vi "field_sweep_0.vi"() -> ()   [LabVIEW 2016]
uses:
  states_field_sweep.ctl
  <vilib>/Utility/error.llb/DialogType.ctl
  <vilib>/DAQmx/write.llb/DAQmx Write (Analog DBL 1Chan 1Samp).vi
  <vilib>/DAQmx/create/channels.llb/DAQmx Create Channel (AO-Voltage-Basic).vi
  <vilib>/DAQmx/miscellaneous.llb/DAQmx Fill In Error Info.vi
  <instrlib>/niVNA/niVNA.llb/niVNA Fetch Sweep Measurement (DBL).vi
panel:
  out "DAQ channel Out":tag="DAQ_6363/ao0"
  in  "Averaging Points":i32=10 min=1 max=3201 step=1
  in  "DAQ channel In":tag="DAQ_6363/ao0"
  in  "Exit Button":bool
  in  "IF Bandwidth":dbl(ring)=1000.0 items=["10 Hz"=10.0, "30 Hz"=30.0, "100 Hz"=100.0, "300 Hz"=300.0, "1 KHz"=1000.0, "3 KHz"=3000.0, "10 KHz"=10000.0, "30 KHz"=30000.0]
  in  "Speed (Oe/sec)":dbl=5.0
  in  "Frequency (Hz)":dbl=3000000000.0 min=10000000.0 max=6000000000.0
  in  "Save Button":bool
  out "Status":string="Shutting down...Sweeping field to zero..."
  out "Cursor":cluster{"x":dbl, "y":dbl} {"x" format="%.2f"; "y" format="%.5f"}
  out "VNA Name Out":refnum<k15>="VNA_5630"
  out "Error Out":errorcluster
  in  "Error In (no error)":errorcluster
  in  "Format":i32(ring)=1 items=["Log Magnitude (dB)"=0, "Lin Magnitude"=1, "Phase (deg)"=2, "VSWR"=3, "Group Delay"=6]
  out "SpectrumGraph":cluster{"Field":dbl[], "Signal":dbl[]}(graph)
  in  "S-parameter":i32(ring)=1 caption="Measurement" items=["S11", "S21"]
  in  "Start Button":bool
  in  "Stop Button":bool
  in  "Output Power (dBm)":dbl=1.0 min=-25.0 max=5.0 step=0.5
  in  "Number of Points":i32=1000 min=1 max=3201 step=1
  in  "Stop H Field (Oe)":dbl=1500.0 min=-6000.0 max=6000.0 format="%#_6f"
  in  "Start H Field (Oe)":dbl=1000.0 min=-6000.0 max=6000.0 format="%#_6f"
  in  "VNA Name In":refnum<k15>="VNA_5630"
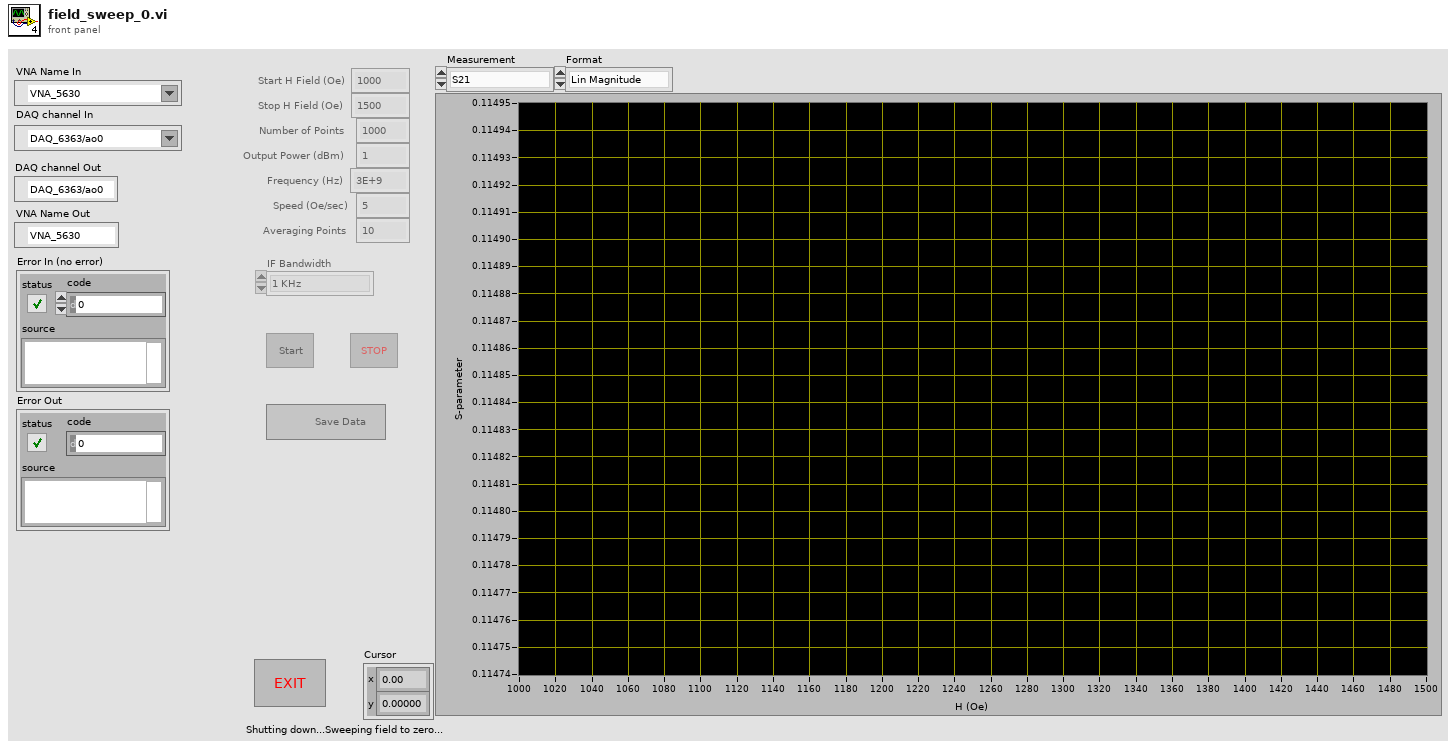
[diagram p1: front panel]
types:
  T1 = typedef "states_field_sweep.ctl" = enum16{"Init", "Idle", "Sweeping up", "Sweeping down", "Running", "Shutdown"}
  T2 = typedef "DialogType.ctl" = u16
  T3 = typedef "LVPoint32TypeDef.ctl" = cluster{"Horizontal":i32, "Vertical":i32}
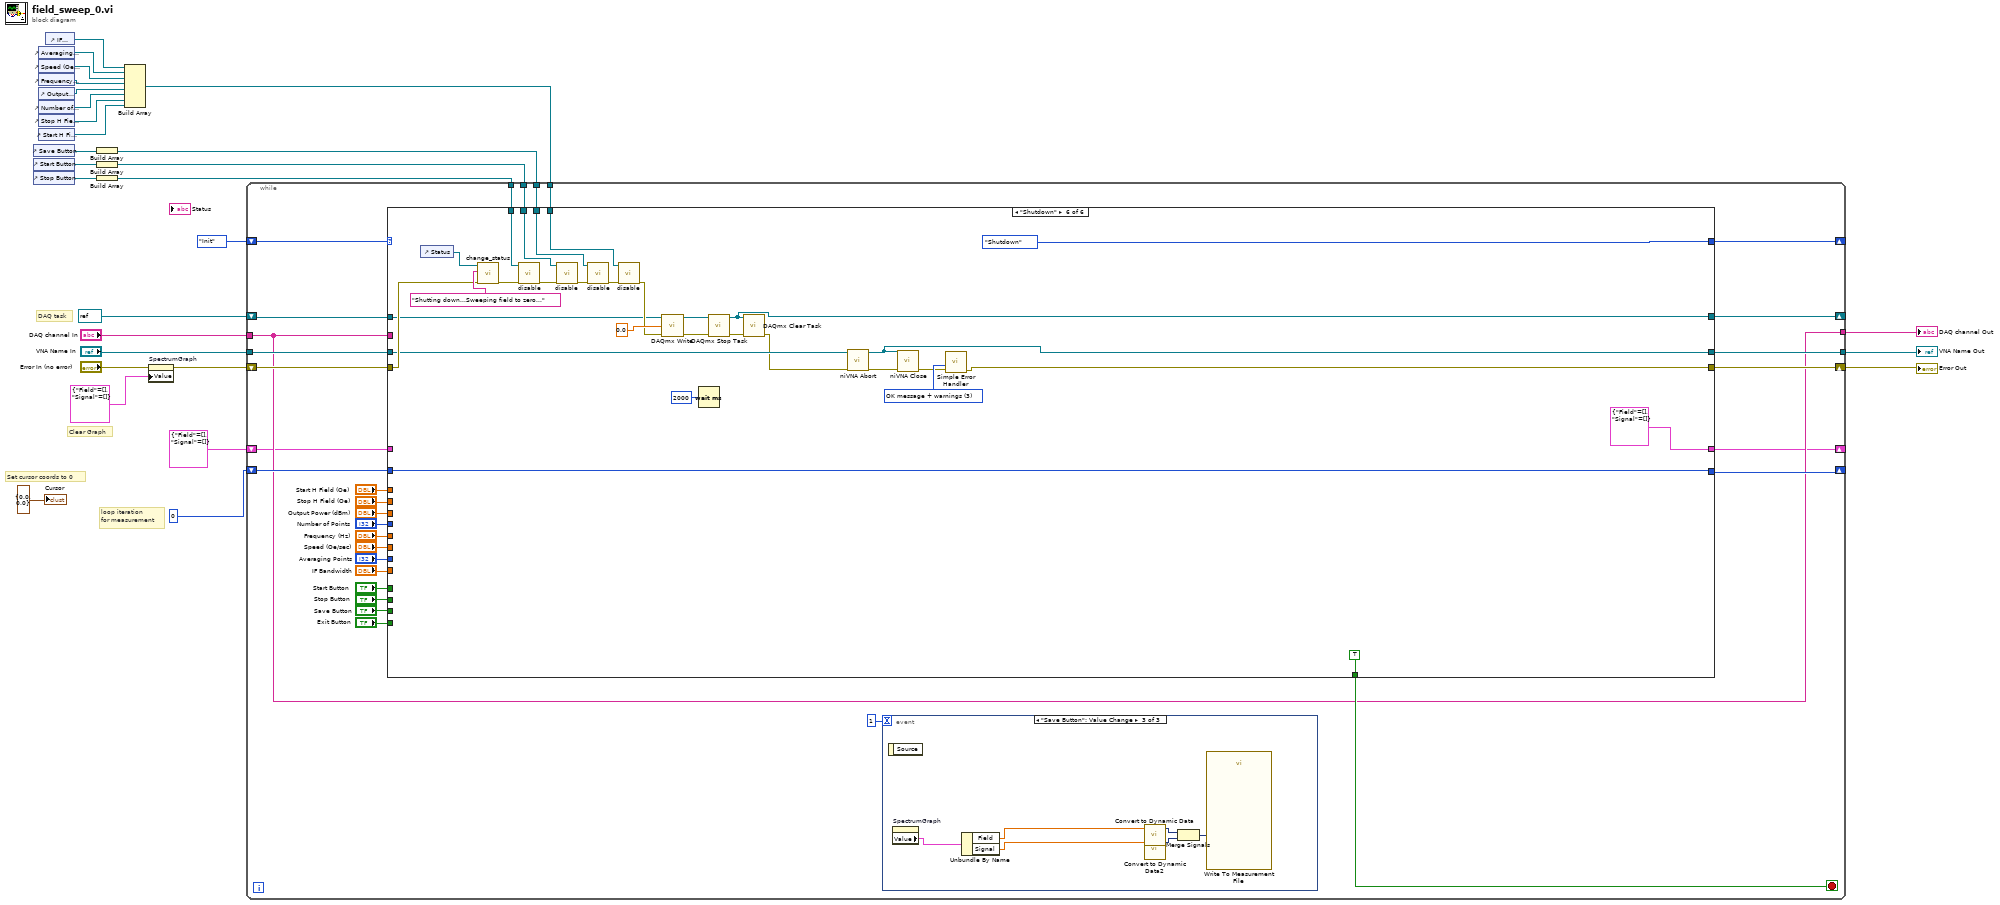
[diagram p0: block diagram]
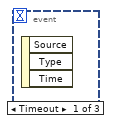
[diagram p2: hidden frame]
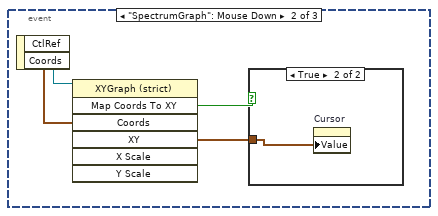
[diagram p3: hidden frame]
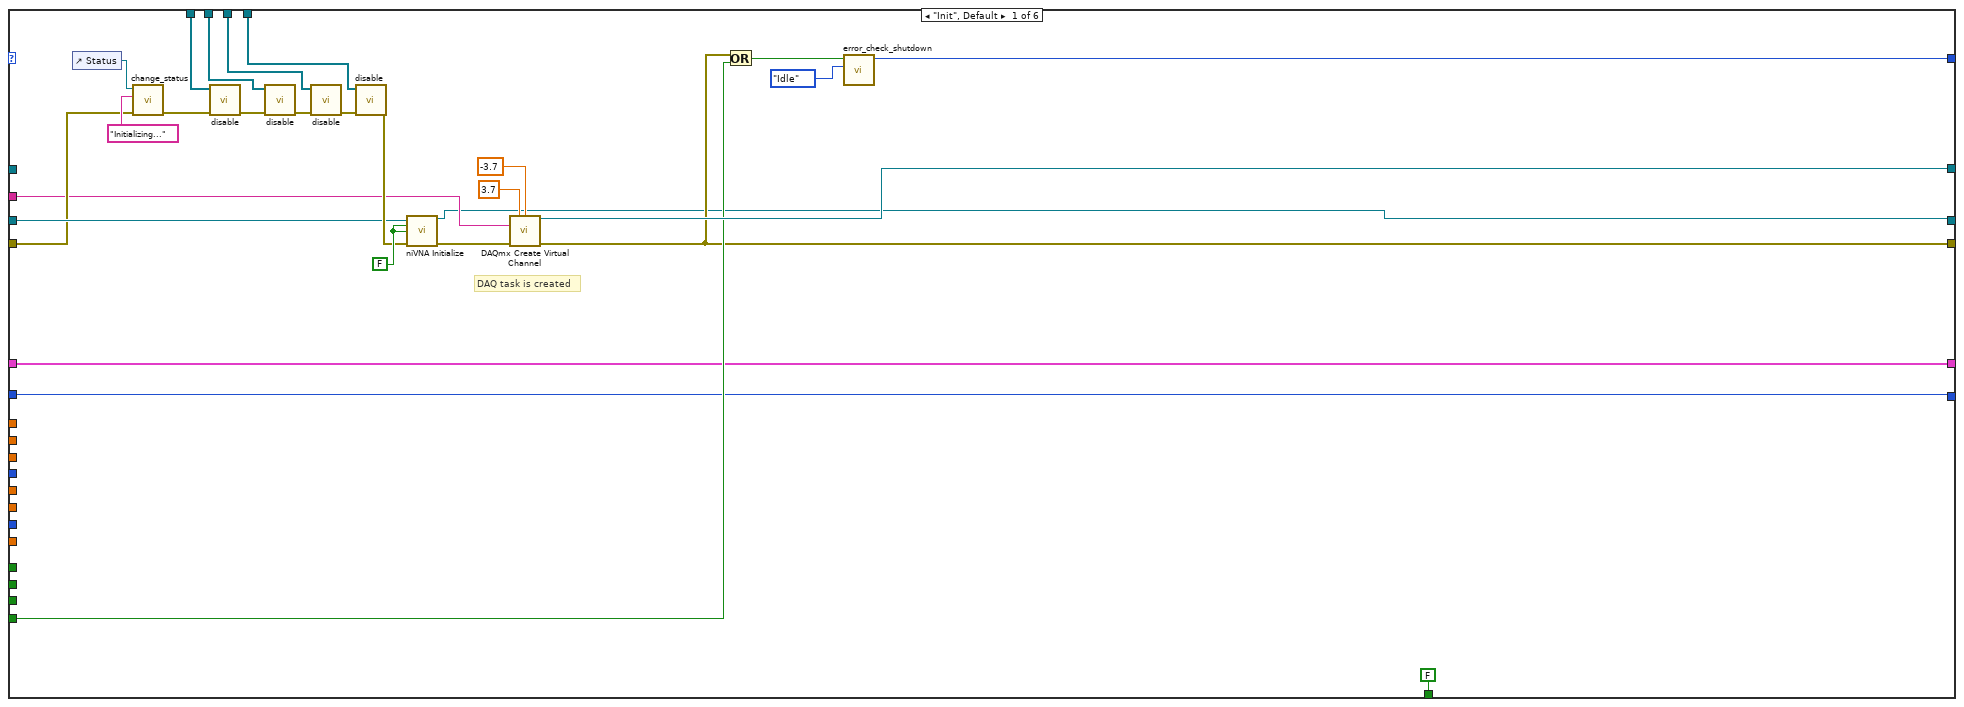
[diagram p5: hidden frame]
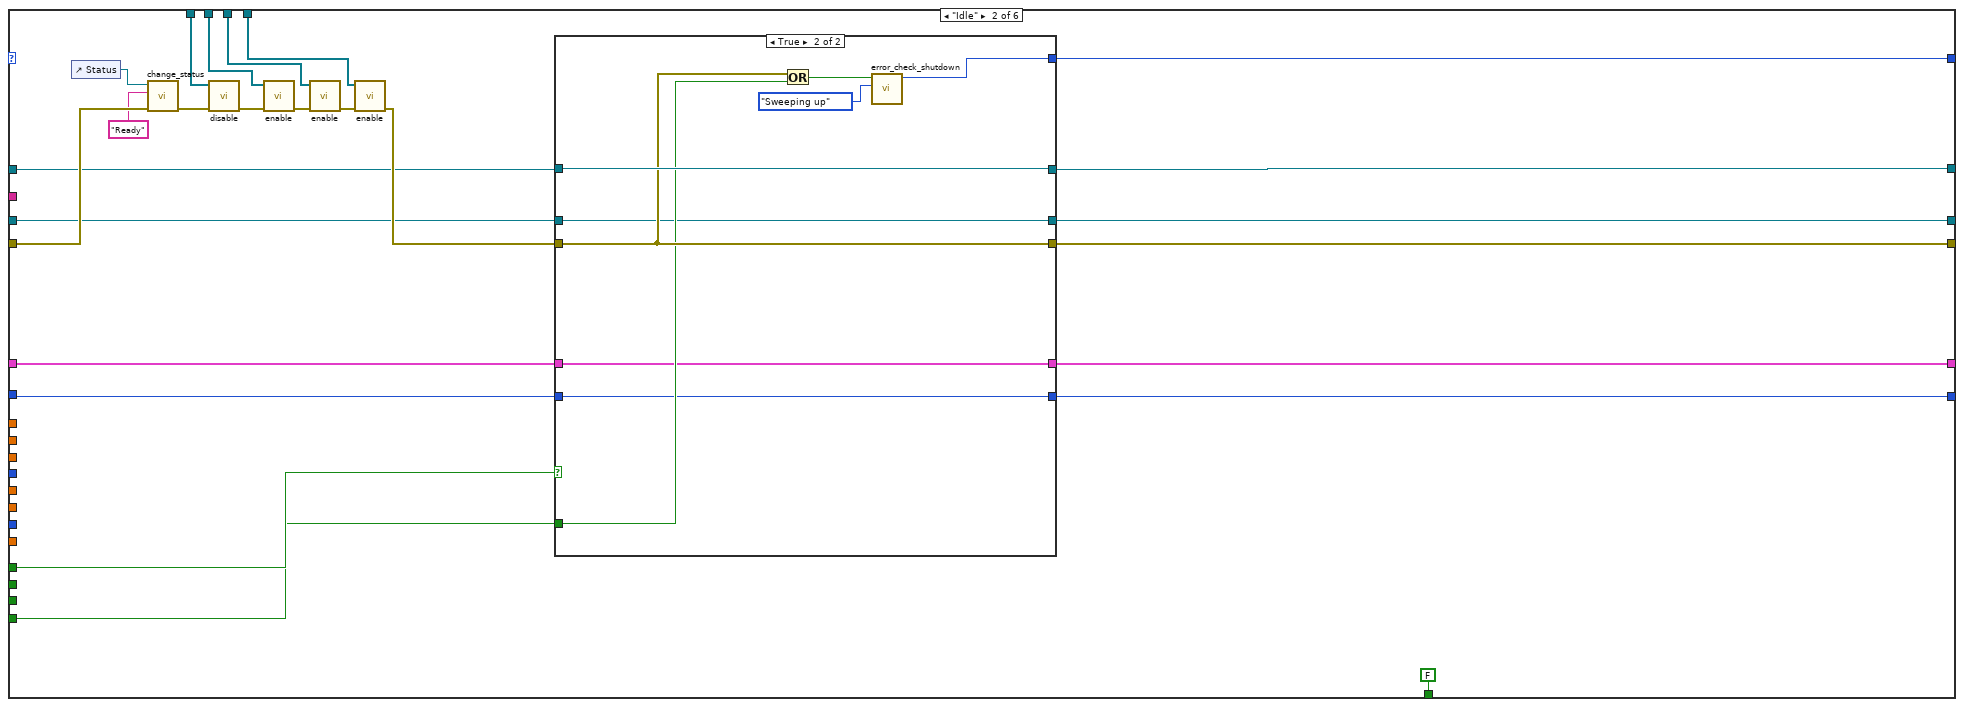
[diagram p6: hidden frame]
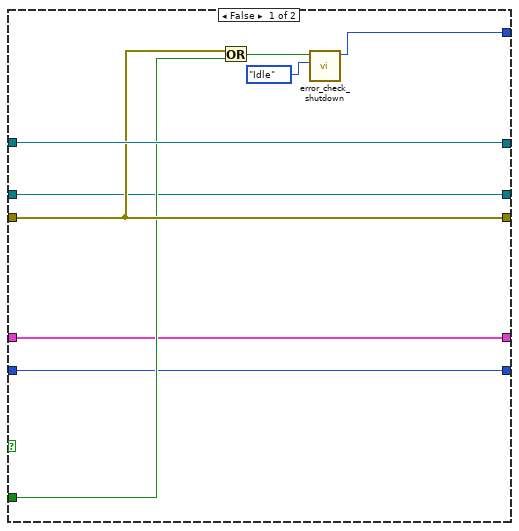
[diagram p7: hidden frame]
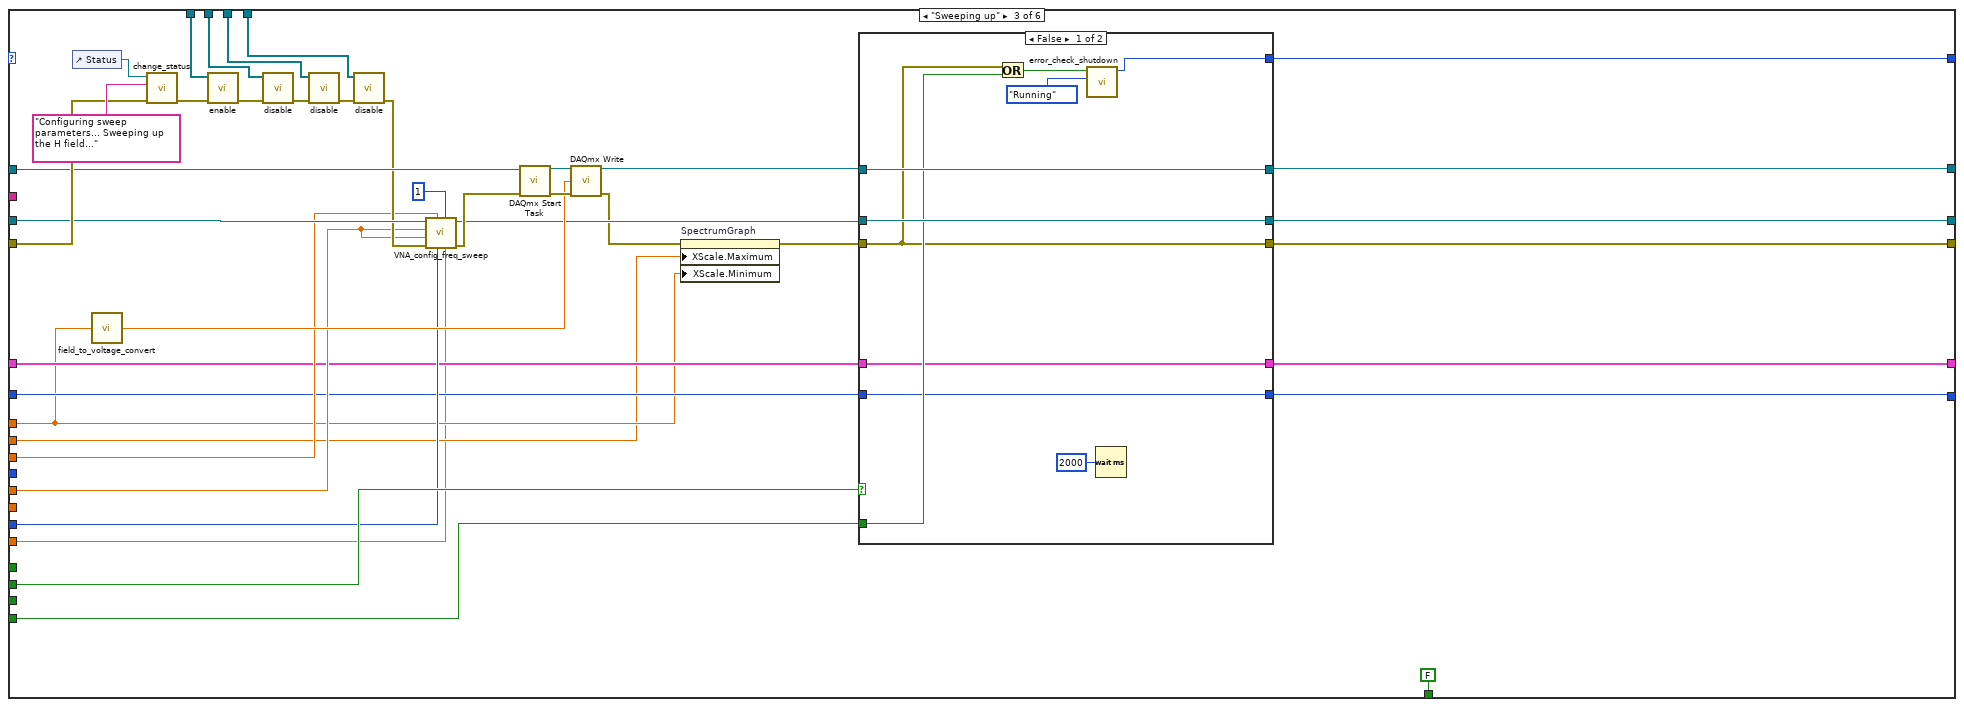
[diagram p8: hidden frame]
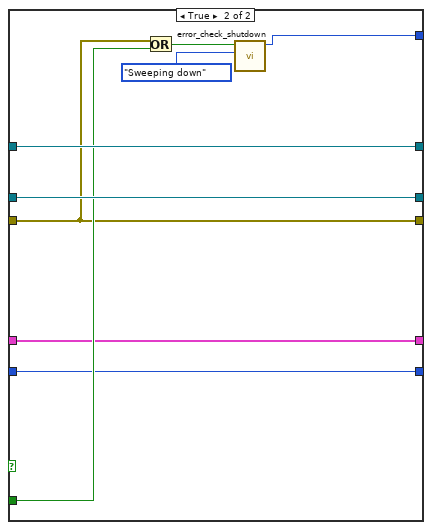
[diagram p9: hidden frame]
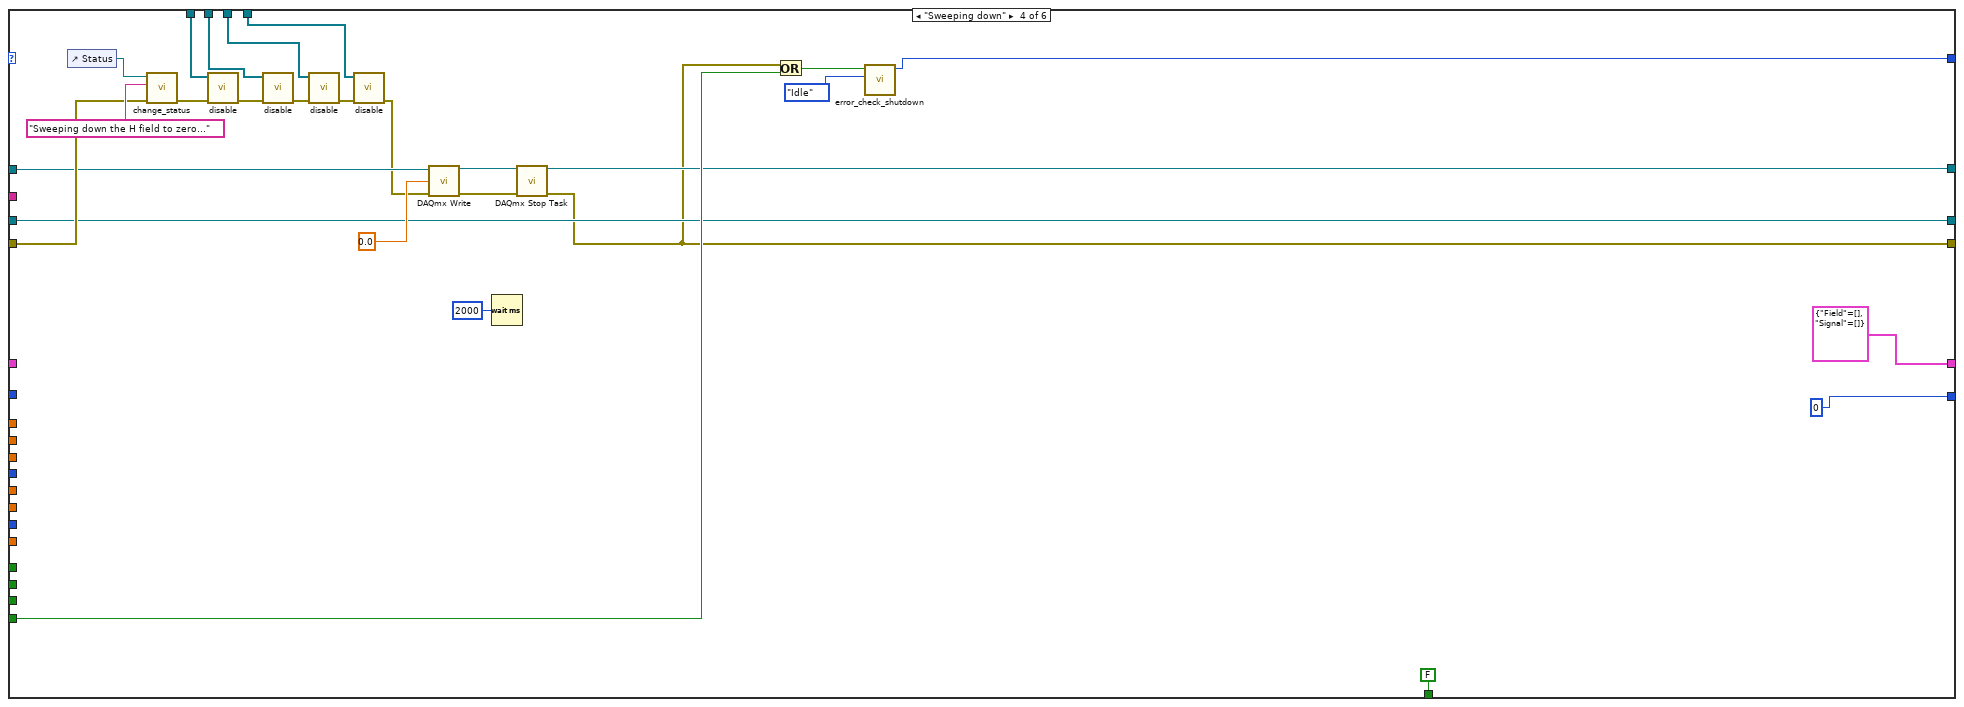
[diagram p10: hidden frame]
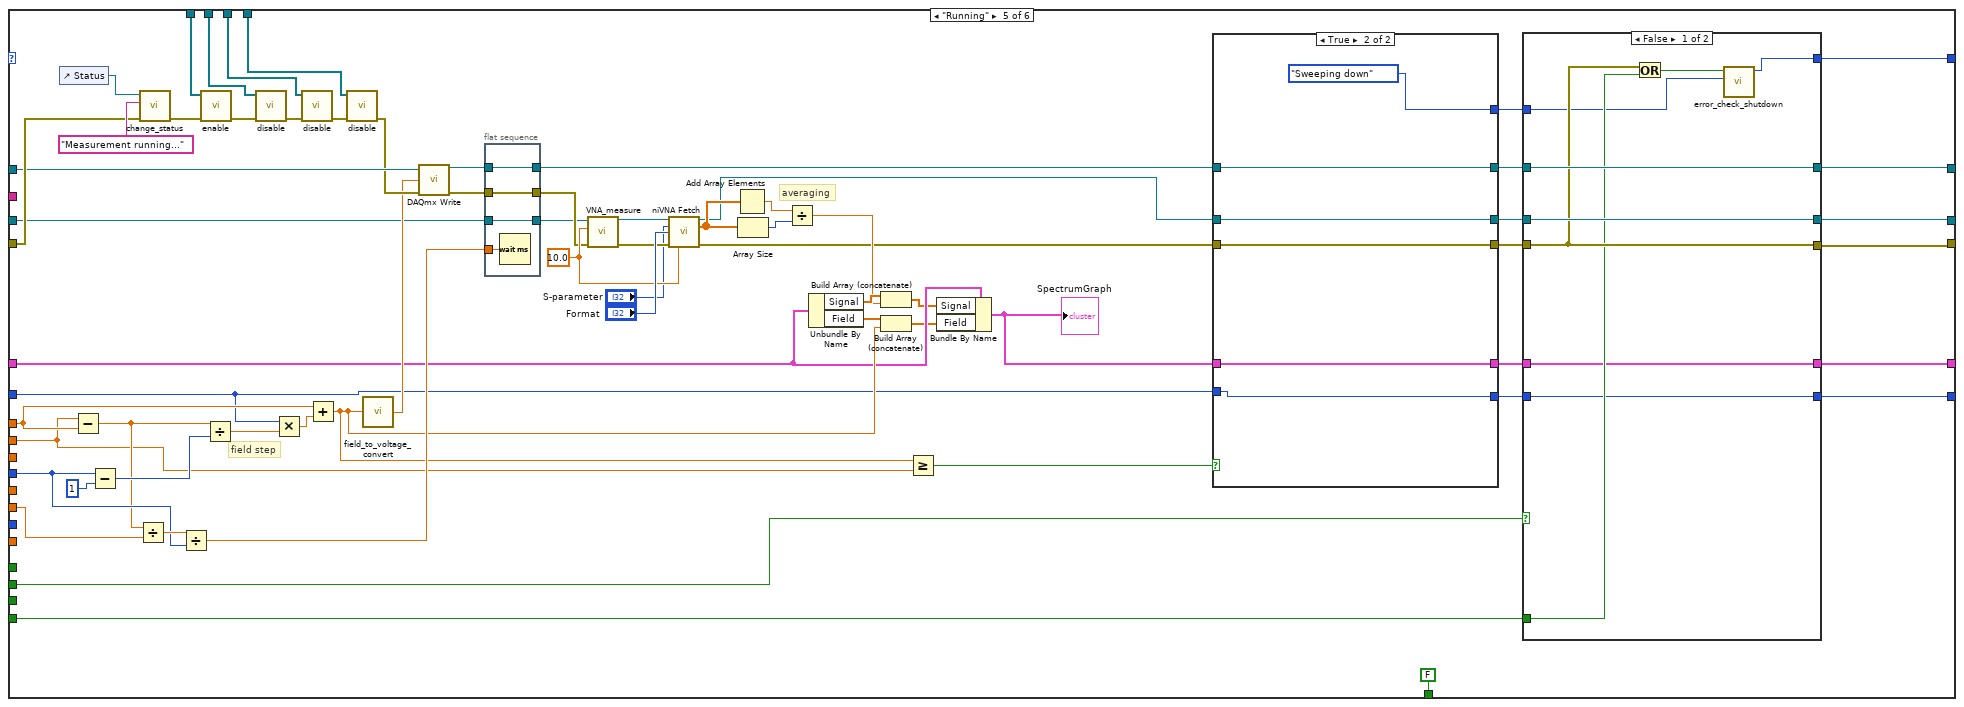
[diagram p11: hidden frame]
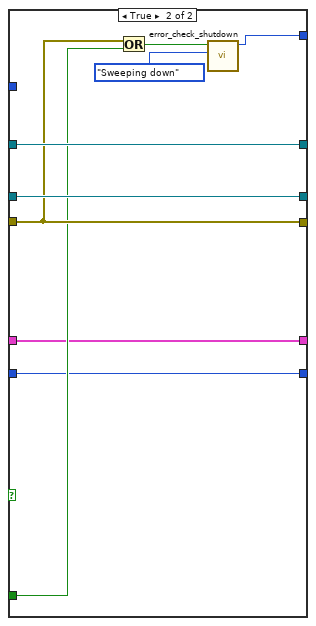
[diagram p12: hidden frame]
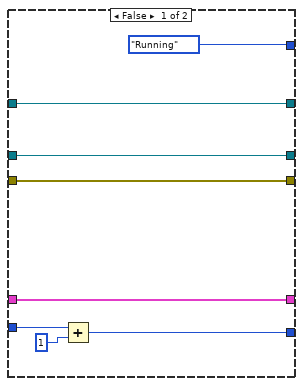
[diagram p13: hidden frame]
diagram:
  # "loop iteration\nfor measurement"
  # "DAQ task"
  # "Set cursor coords to 0"
  # "Clear Graph"
  n1 = control-ref of="Save Button"() -> (w11:refnum<vi>)
  n2 = control-ref of="Start Button"() -> (w19:refnum<vi>)
  n3 = control-ref of="Stop Button"() -> (w18:refnum<vi>)
  n4 = control-ref of="Averaging Points"() -> (w8:refnum<vi>)
  n5 = control-ref of="Speed (Oe/sec)"() -> (w25:refnum<vi>)
  n6 = control-ref of="Frequency (Hz)"() -> (w24:refnum<vi>)
  n7 = control-ref of="Output Power (dBm)"() -> (w23:refnum<vi>)
  n8 = control-ref of="Number of Points"() -> (w22:refnum<vi>)
  n9 = control-ref of="Stop H Field (Oe)"() -> (w21:refnum<vi>)
  n10 = control-ref of="Start H Field (Oe)"() -> (w20:refnum<vi>)
  n11 = control-ref of="IF Bandwidth"() -> (w26:refnum<vi>)
  n12 = Build Array(w11) -> (w10:refnum<vi>[])
  n13 = Build Array(w19) -> (w16:refnum<vi>[])
  n14 = Build Array(w18) -> (w15:refnum<vi>[])
  n15 = Build Array(w26, w8, w25, w24, w23, w22, w21, w20) -> (w17:refnum<vi>[])
  n16 = property on="SpectrumGraph" class="XYGraph (strict)"(error in="Error In (no error)", "Value"=cluster{"Field":dbl[], "Signal":dbl[]} {"Field"=[], "Signal"=[]} ("SpectrumGraph")) -> (error out=w3:errorcluster)  [unwired: 1 in, 1 out]
  n17 = while {
    shift-right: [w54] -> _
    shift-left: states_field_sweep."Init" -> [w59]
    shift-right: [w34] -> _
    shift-left: 0 -> [w36]
    tunnel: w17 -> [w58]
    tunnel: w16 -> [w57]
    tunnel: w15 -> [w56]
    tunnel: "VNA Name In" -> [w55]
    tunnel: "DAQ channel In" -> [w33]
    shift-right: [w53] -> w7
    shift-left: w3 -> [w52]
    shift-right: [w51] -> _
    shift-left: refnum<k21> refnum ("task in") -> [w50]
    tunnel: w10 -> [w49]
    tunnel: [w37] -> w6
    shift-right: [w29] -> _
    shift-left: cluster{"Field":dbl[], "Signal":dbl[]} {"Field"=[], "Signal"=[]} -> [w30]
    tunnel: [w33] -> w5
    stop <- w44 stop-if-true
    n18 = case shown="\"Shutdown\"" w59 {
      tunnel: w58 -> [w82 w120 w173 w218 w285 w350]
      tunnel: w57 -> [w96 w122 w175 w216 w287 w352]
      tunnel: w56 -> [w98 w123 w176 w215 w289 w353]
      tunnel: w55 -> [w90 w109 w159 w210 w251 w334]
      tunnel: w52 -> [w89 w115 w171 w222 w283 w348]
      tunnel: [w77 w106 w161 w211 w234 states_field_sweep."Shutdown"] -> w54
      tunnel: w33 -> [w85 _ _ _ _ _]
      tunnel: [w76 w110 w169 w203 w241 w343] -> w53
      tunnel: [w84 w107 w167 w205 w245 w344] -> w51
      tunnel: w50 -> [_ w108 w166 w220 w282 w337]
      tunnel: w49 -> [w83 w121 w174 w217 w286 w351]
      tunnel: "Start Button" -> [_ w112 _ _ _ _]
      tunnel: "Stop Button" -> [_ _ w170 _ w240 _]
      tunnel: "Save Button" -> [_ _ _ _ _ _]
      tunnel: "Exit Button" -> [w79 w105 w160 w212 w239 _]
      tunnel: [FALSE FALSE FALSE FALSE FALSE TRUE] -> w44
      tunnel: "Start H Field (Oe)" -> [_ _ w146 _ w261 _]
      tunnel: "Stop H Field (Oe)" -> [_ _ w145 _ w254 _]
      tunnel: "Output Power (dBm)" -> [_ _ w154 _ _ _]
      tunnel: "Number of Points" -> [_ _ _ _ w266 _]
      tunnel: "Frequency (Hz)" -> [_ _ w155 _ _ _]
      tunnel: "Speed (Oe/sec)" -> [_ _ _ _ w268 _]
      tunnel: [w74 w104 w168 w210 w243 w345] -> w37
      tunnel: w36 -> [w73 w101 w151 _ w247 w331]
      tunnel: "Averaging Points" -> [_ _ w153 _ _ _]
      tunnel: w30 -> [w71 w103 w152 _ w232 _]
      tunnel: [w73 w102 w150 0 w236 w331] -> w34
      tunnel: "IF Bandwidth" -> [_ _ w144 _ _ _]
      tunnel: [w71 w99 w143 cluster{"Field":dbl[], "Signal":dbl[]} {"Field"=[], "Signal"=[]} w228 cluster{"Field":dbl[], "Signal":dbl[]} {"Field"=[], "Signal"=[]}] -> w29
      frame "Init", Default {
        w92 = FALSE ("id query")
        # "DAQ task is created"
        n19 = control-ref of="Status"() -> (w94:refnum<vi>)
        n20 = call "change_status.vi"("error in (no error)"=w89, "String"="Initializing...", "String in"=w94) -> ("error out"=w95:errorcluster)  [unwired: 8 in]
        n21 = call "disable.vi"("error in (no error)"=w95, "Array"=w98) -> ("error out"=w97:errorcluster)  [unwired: 9 in]
        n22 = call "disable.vi"("error in (no error)"=w97, "Array"=w96) -> ("error out"=w81:errorcluster)  [unwired: 9 in]
        n23 = call "disable.vi"("error in (no error)"=w81, "Array"=w83) -> ("error out"=w80:errorcluster)  [unwired: 9 in]
        n24 = call "disable.vi"("error in (no error)"=w80, "Array"=w82) -> ("error out"=w91:errorcluster)  [unwired: 9 in]
        n25 = call <instrlib>:"niVNA Initialize.vi"("resource name"=w90, "id query"=w92, "reset"=w92, "error in"=w91) -> ("instrument handle"=w74:refnum<k15>, "error out"=w88:errorcluster)  [unwired: 10 in]
        n26 = call-poly <vilib>:"DAQmx Create Virtual Channel.vi"("maximum value"=3.7, "minimum value"=-3.7, "physical channels"=w85, "error in"=w88) -> ("task out"=w84:refnum<k21>, "error out"=w76:errorcluster)  [unwired: 10 in]
        n27 = Or(x=w76, y=w79) -> (x .or. y?=w75:bool)
        n28 = call "error_check_shutdown.vi"("Enum in"=states_field_sweep."Idle", "Boolean"=w75) -> ("Enum out"=w77:T1)  [unwired: 9 in]
      }
      frame "Idle" {
        n29 = control-ref of="Status"() -> (w114:refnum<vi>)
        n30 = call "change_status.vi"("error in (no error)"=w115, "String"="Ready", "String in"=w114) -> ("error out"=w116:errorcluster)  [unwired: 8 in]
        n31 = call "disable.vi"("error in (no error)"=w116, "Array"=w123) -> ("error out"=w119:errorcluster)  [unwired: 9 in]
        n32 = call "enable.vi"("error in (no error)"=w119, "Array"=w122) -> ("error out"=w118:errorcluster)  [unwired: 9 in]
        n33 = call "enable.vi"("error in (no error)"=w118, "Array"=w121) -> ("error out"=w117:errorcluster)  [unwired: 9 in]
        n34 = call "enable.vi"("error in (no error)"=w117, "Array"=w120) -> ("error out"=w111:errorcluster)  [unwired: 9 in]
        n35 = case shown="True" w112 {
          tunnel: w111 -> [w128 w138]
          tunnel: [w128 w138] -> w110
          tunnel: w109 -> [w126 w135]
          tunnel: w108 -> [w132 w141]
          tunnel: [w132 w141] -> w107
          tunnel: [w129 w136] -> w106
          tunnel: w105 -> [w127 w137]
          tunnel: [w126 w135] -> w104
          tunnel: w103 -> [w125 w134]
          tunnel: [w125 w134] -> w99
          tunnel: [w124 w133] -> w102
          tunnel: w101 -> [w124 w133]
          frame False {
            n36 = Or(x=w128, y=w127) -> (x .or. y?=w130:bool)
            n37 = call "error_check_shutdown.vi"("Enum in"=states_field_sweep."Idle", "Boolean"=w130) -> ("Enum out"=w129:T1)  [unwired: 9 in]
          }
          frame True {
            n38 = Or(x=w138, y=w137) -> (x .or. y?=w139:bool)
            n39 = call "error_check_shutdown.vi"("Enum in"=states_field_sweep."Sweeping up", "Boolean"=w139) -> ("Enum out"=w136:T1)  [unwired: 9 in]
          }
        }
      }
      frame "Sweeping up" {
        n40 = control-ref of="Status"() -> (w172:refnum<vi>)
        n41 = call "field_to_voltage_convert.vi"("Start H Field (Oe)"=w146) -> ("Numeric"=w162:dbl)
        n42 = call "change_status.vi"("error in (no error)"=w171, "String"="Configuring sweep parameters... Sweeping up the H field...", "String in"=w172) -> ("error out"=w180:errorcluster)  [unwired: 8 in]
        n43 = call "enable.vi"("error in (no error)"=w180, "Array"=w176) -> ("error out"=w179:errorcluster)  [unwired: 9 in]
        n44 = call "disable.vi"("error in (no error)"=w179, "Array"=w175) -> ("error out"=w178:errorcluster)  [unwired: 9 in]
        n45 = call "disable.vi"("error in (no error)"=w178, "Array"=w174) -> ("error out"=w177:errorcluster)  [unwired: 9 in]
        n46 = call "disable.vi"("error in (no error)"=w177, "Array"=w173) -> ("error out"=w158:errorcluster)  [unwired: 9 in]
        n47 = call "VNA_config_freq_sweep.vi"("IF Bandwidth"=w144, "Averaging"=1, "Number of Points"=w153, "Output Power"=w154, "error in (no error)"=w158, "Stop Frequency"=w155, "Start Frequency"=w155, "Resource Name In"=w159) -> ("error out"=w157:errorcluster, "Resource Name Out"=w156:refnum<k15>)  [unwired: 2 in]
        n48 = call <vilib>:"DAQmx Start Task.vi"("task/channels in"=w166, "error in"=w157) -> ("task out"=w165:refnum<k21>, "error out"=w163:errorcluster)  [unwired: 12 in]
        n49 = call-poly <vilib>:"DAQmx Write.vi"("task/channels in"=w165, "data"=w162, "error in"=w163) -> ("task out"=w164:refnum<k21>, "error out"=w148:errorcluster)  [unwired: 10 in, 1 out]
        n50 = property on="SpectrumGraph" class="XYGraph (strict)"(error in=w148, "XScale.Maximum"=w145, "XScale.Minimum"=w146) -> (error out=w147:errorcluster)  [unwired: 1 in, 1 out]
        n51 = case shown="False" w170 {
          tunnel: w147 -> [w185 w194]
          tunnel: w164 -> [w191 w199]
          tunnel: w156 -> [w190 w200]
          tunnel: [w185 w194] -> w169
          tunnel: [w190 w200] -> w168
          tunnel: [w191 w199] -> w167
          tunnel: [w187 w196] -> w161
          tunnel: w160 -> [w186 w195]
          tunnel: w152 -> [w183 w193]
          tunnel: [w183 w193] -> w143
          tunnel: w151 -> [w182 w192]
          tunnel: [w182 w192] -> w150
          frame False {
            n52 = Or(x=w185, y=w186) -> (x .or. y?=w188:bool)
            n53 = call "error_check_shutdown.vi"("Enum in"=states_field_sweep."Running", "Boolean"=w188) -> ("Enum out"=w187:T1)  [unwired: 9 in]
            n54 = Wait (ms)(milliseconds to wait=u32 2000) -> ()  [unwired: 1 out]
          }
          frame True {
            n55 = Or(x=w194, y=w195) -> (x .or. y?=w197:bool)
            n56 = call "error_check_shutdown.vi"("Enum in"=states_field_sweep."Sweeping down", "Boolean"=w197) -> ("Enum out"=w196:T1)  [unwired: 9 in]
          }
        }
      }
      frame "Sweeping down" {
        n57 = control-ref of="Status"() -> (w209:refnum<vi>)
        n58 = call "change_status.vi"("error in (no error)"=w222, "String"="Sweeping down the H field to zero...", "String in"=w209) -> ("error out"=w226:errorcluster)  [unwired: 8 in]
        n59 = call "disable.vi"("error in (no error)"=w226, "Array"=w215) -> ("error out"=w225:errorcluster)  [unwired: 9 in]
        n60 = call "disable.vi"("error in (no error)"=w225, "Array"=w216) -> ("error out"=w224:errorcluster)  [unwired: 9 in]
        n61 = call "disable.vi"("error in (no error)"=w224, "Array"=w217) -> ("error out"=w223:errorcluster)  [unwired: 9 in]
        n62 = call "disable.vi"("error in (no error)"=w223, "Array"=w218) -> ("error out"=w219:errorcluster)  [unwired: 9 in]
        n63 = call-poly <vilib>:"DAQmx Write.vi"("task/channels in"=w220, "data"=0.0, "error in"=w219) -> ("task out"=w206:refnum<k21>, "error out"=w204:errorcluster)  [unwired: 10 in, 1 out]
        n64 = Wait (ms)(milliseconds to wait=u32 2000) -> ()  [unwired: 1 out]
        n65 = call <vilib>:"DAQmx Stop Task.vi"("task/channels in"=w206, "error in"=w204) -> ("task out"=w205:refnum<k21>, "error out"=w203:errorcluster)  [unwired: 12 in]
        n66 = Or(x=w203, y=w212) -> (x .or. y?=w213:bool)
        n67 = call "error_check_shutdown.vi"("Enum in"=states_field_sweep."Idle", "Boolean"=w213) -> ("Enum out"=w211:T1)  [unwired: 9 in]
      }
      frame "Running" {
        w275 = 10.0 ("timeout")
        # "averaging"
        # "field step"
        n68 = control-ref of="Status"() -> (w284:refnum<vi>)
        n69 = Subtract(x=w254, y=w261) -> (x-y=w259:dbl)
        n70 = Subtract(x=w266, y=1) -> (x-y=w279:i32)
        n71 = Divide(x=w259, y=w268) -> (x/y=w267:dbl)
        n72 = call "change_status.vi"("error in (no error)"=w283, "String"="Measurement running...", "String in"=w284) -> ("error out"=w290:errorcluster)  [unwired: 8 in]
        n73 = Divide(x=w267, y=w266) -> (x/y=w265:dbl)
        n74 = call "enable.vi"("error in (no error)"=w290, "Array"=w289) -> ("error out"=w293:errorcluster)  [unwired: 9 in]
        n75 = Divide(x=w259, y=w279) -> (x/y=w278:dbl)
        n76 = call "disable.vi"("error in (no error)"=w293, "Array"=w287) -> ("error out"=w292:errorcluster)  [unwired: 9 in]
        n77 = Multiply(x=w247, y=w278) -> (x*y=w277:dbl)
        n78 = call "disable.vi"("error in (no error)"=w292, "Array"=w286) -> ("error out"=w291:errorcluster)  [unwired: 9 in]
        n79 = Add(x=w261, y=w277) -> (x+y=w255:dbl)
        n80 = call "disable.vi"("error in (no error)"=w291, "Array"=w285) -> ("error out"=w281:errorcluster)  [unwired: 9 in]
        n81 = call "field_to_voltage_convert.vi"("Start H Field (Oe)"=w255) -> ("Numeric"=w260:dbl)
        n82 = call-poly <vilib>:"DAQmx Write.vi"("task/channels in"=w282, "data"=w260, "error in"=w281) -> ("task out"=w264:refnum<k21>, "error out"=w263:errorcluster)  [unwired: 10 in, 1 out]
        n83 = flat-sequence {
          tunnel: w265 -> [w329]
          tunnel: w264 -> [w328]
          tunnel: [w328] -> w252
          tunnel: w263 -> [w327]
          tunnel: [w327] -> w262
          tunnel: w251 -> [w326]
          tunnel: [w326] -> w250
          frame #0 {
            n84 = Wait (ms)(milliseconds to wait=w329) -> ()  [unwired: 1 out]
          }
        }
        n85 = call "VNA_measure.vi"("error in (no error)"=w262, "timeout"=w275, "Resource Name In"=w250) -> ("error out"=w274:errorcluster, "Resource Name Out"=w272:refnum<k15>)  [unwired: 7 in]
        n86 = call-poly <instrlib>:"niVNA Fetch.vi"("instrument handle"=w272, "measurement"="S-parameter", "format"="Format", "error in"=w274, "timeout"=w275) -> ("instrument handle out"=w249:refnum<k15>, "data"=w271:dbl[], "error out"=w248:errorcluster)  [unwired: 7 in, 1 out]
        n87 = Add Array Elements(numeric array=w271) -> (sum=w270:dbl)
        n88 = Array Size(array=w271) -> (size(s)=w269:i32)
        n89 = Divide(x=w270, y=w269) -> (x/y=w257:dbl)
        n90 = Unbundle By Name(w232) -> ("Signal"=w258:dbl[], "Field"=w256:dbl[])
        n91 = Build Array (concatenate)(w258, w257) -> (w231:dbl[])
        n92 = Build Array (concatenate)(w256, w255) -> (w230:dbl[])
        n93 = Greater Or Equal?(x=w255, y=w254) -> (x >= y?=w253:bool)
        n94 = Bundle By Name(cluster=w232, "Signal"=w231, "Field"=w230) -> (w229:cluster{"Field":dbl[], "Signal":dbl[]})
        "SpectrumGraph" <- w229
        n95 = case shown="True" w253 {
          tunnel: w229 -> [w319 w320]
          tunnel: [w319 w320] -> w238
          tunnel: [states_field_sweep."Running" states_field_sweep."Sweeping down"] -> w235
          tunnel: w252 -> [w317 w323]
          tunnel: [w317 w323] -> w246
          tunnel: w249 -> [w316 w324]
          tunnel: [w316 w324] -> w244
          tunnel: w248 -> [w315 w322]
          tunnel: [w315 w322] -> w242
          tunnel: w247 -> [w314 w321]
          tunnel: [w312 w321] -> w237
          frame False {
            n96 = Add(x=w314, y=1) -> (x+y=w312:i32)
          }
          frame True {
          }
        }
        n97 = case shown="False" w240 {
          tunnel: [w301 w309] -> w234
          tunnel: w246 -> [w300 w308]
          tunnel: [w300 w308] -> w245
          tunnel: w244 -> [w299 w307]
          tunnel: [w299 w307] -> w243
          tunnel: w242 -> [w298 w306]
          tunnel: [w298 w306] -> w241
          tunnel: w239 -> [w297 w305]
          tunnel: w238 -> [w296 w304]
          tunnel: [w296 w304] -> w228
          tunnel: w237 -> [w295 w303]
          tunnel: [w295 w303] -> w236
          tunnel: w235 -> [w294 _]
          frame False {
            n98 = Or(x=w298, y=w297) -> (x .or. y?=w302:bool)
            n99 = call "error_check_shutdown.vi"("Enum in"=w294, "Boolean"=w302) -> ("Enum out"=w301:T1)  [unwired: 9 in]
          }
          frame True {
            n100 = Or(x=w306, y=w305) -> (x .or. y?=w310:bool)
            n101 = call "error_check_shutdown.vi"("Enum in"=states_field_sweep."Sweeping down", "Boolean"=w310) -> ("Enum out"=w309:T1)  [unwired: 9 in]
          }
        }
      }
      frame "Shutdown" {
        w342 = T2 3 items=["no dialog", "OK message", "continue or stop message", "OK message + warnings", "continue/stop + warnings"] ("type of dialog (OK msg:1)")
        n102 = control-ref of="Status"() -> (w349:refnum<vi>)
        n103 = call "change_status.vi"("error in (no error)"=w348, "String"="Shutting down...Sweeping field to zero...", "String in"=w349) -> ("error out"=w355:errorcluster)  [unwired: 8 in]
        n104 = call "disable.vi"("error in (no error)"=w355, "Array"=w353) -> ("error out"=w358:errorcluster)  [unwired: 9 in]
        n105 = call "disable.vi"("error in (no error)"=w358, "Array"=w352) -> ("error out"=w357:errorcluster)  [unwired: 9 in]
        n106 = call "disable.vi"("error in (no error)"=w357, "Array"=w351) -> ("error out"=w356:errorcluster)  [unwired: 9 in]
        n107 = call "disable.vi"("error in (no error)"=w356, "Array"=w350) -> ("error out"=w338:errorcluster)  [unwired: 9 in]
        n108 = call-poly <vilib>:"DAQmx Write.vi"("task/channels in"=w337, "data"=0.0, "error in"=w338) -> ("task out"=w335:refnum<k21>, "error out"=w336:errorcluster)  [unwired: 10 in, 1 out]
        n109 = Wait (ms)(milliseconds to wait=u32 2000) -> ()  [unwired: 1 out]
        n110 = call <vilib>:"DAQmx Stop Task.vi"("task/channels in"=w335, "error in"=w336) -> ("task out"=w344:refnum<k21>, "error out"=w346:errorcluster)  [unwired: 12 in]
        n111 = call <vilib>:"DAQmx Clear Task.vi"("task in"=w344, "error in"=w346) -> ("error out"=w333:errorcluster)  [unwired: 13 in]
        n112 = call <instrlib>:"niVNA Abort.vi"("instrument handle"=w334, "error in"=w333) -> ("instrument handle out"=w345:refnum<k15>, "error out"=w347:errorcluster)  [unwired: 12 in]
        n113 = call <instrlib>:"niVNA Close.vi"("instrument handle"=w345, "error in"=w347) -> ("error out"=w332:errorcluster)  [unwired: 13 in]
        n114 = call <vilib>:"Simple Error Handler.vi"("type of dialog (OK msg:1)"=w342, "error in (no error)"=w332) -> ("error out"=w343:errorcluster)  [unwired: 3 in, 4 out]
      }
    }
    n115 = event shown="[2] \"Save Button\": Value Change" {
      selector: _ -> [_ _ _]
      dyn-events: _ -> [_ _ _]
      timeout: 1 -> [_ _ _]
      event Timeout {
        n116 = event-data() -> ()  [unwired: 1 in, 3 out]
      }
      event "SpectrumGraph": Mouse Down {
        n117 = event-data() -> ("CtlRef"=w60:refnum<vi>, "Coords"=w61:T3)  [unwired: 1 in]
        n118 = invoke on="Invoke Node" class="XYGraph (strict)" method="Map Coords To XY"(reference=w60, "Coords"=w61) -> ("Map Coords To XY"=w62:bool, "XY"=w63:cluster{"X":dbl, "Y":dbl})  [unwired: 5 in, 5 out]
        n119 = case shown="True" w62 {
          tunnel: w63 -> [_ w64]
          frame False {
          }
          frame True {
            n120 = property on="Cursor" class="Clust (strict)"("Value"=w64) -> ()  [unwired: 2 in, 2 out]
          }
        }
      }
      event "Save Button": Value Change {
        n121 = event-data() -> ()  [unwired: 1 in, 1 out]
        n122 = property on="SpectrumGraph" class="XYGraph (strict)"() -> ("Value"=w65:cluster{"Field":dbl[], "Signal":dbl[]})  [unwired: 2 in, 2 out]
        n123 = Unbundle By Name(w65) -> ("Field"=w67:dbl[], "Signal"=w66:dbl[])
        n124 = call "Convert to Dynamic Data"("Array"=w67) -> ("Dynamic Data Type"=w70:dynamicdata)  [unwired: 3 in]
        n125 = call "Convert to Dynamic Data2"("Array"=w66) -> ("Dynamic Data Type"=w68:dynamicdata)  [unwired: 3 in]
        n126 = Merge Signals(w70, w68) -> (w69:dynamicdata)
        n127 = call "Write To Measurement File"("Signals"=w69) -> ()  [unwired: 16 in, 3 out]
      }
    }
  }
  "Error Out" <- w7
  "VNA Name Out" <- w6
  "DAQ channel Out" <- w5
  "Cursor" <- cluster{"x":dbl, "y":dbl} {"x"=0.0, "y"=0.0} ("Cursor")
